vi "VI_WithXControl.vi"(11 "Min Max Slider XControl":dbl(xcontrol)=-inf) -> (3 "Min Max Slider XControl 2":dbl(xcontrol)=-inf)   [LabVIEW 2012]
uses:
  Min Max Slider XControl.xctl
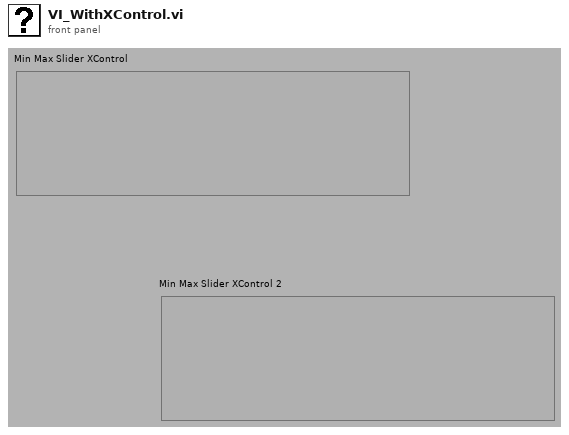
[diagram p1: front panel]
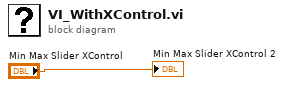
[diagram p0: block diagram]
diagram:
  "Min Max Slider XControl 2" <- "Min Max Slider XControl"
